vi "Status System State.vi"(5 "Retry Attempts (0)":i32 min=0, 7 "Unit Address (-1)":i32=-1, 8 "error in (no error)":errorcluster, 11 "VISA resource name (in)":refnum<visa-resource-name>) -> (0 "error out":errorcluster, 2 "System State":T1, 3 "VISA resource name (out)":refnum<visa-resource-name>)   [LabVIEW 2020, in "Omega Platinum Series.lvlib"]
doc: "Checks the current System State of the controller."
uses:
  <instrlib>/RxnRover/OmegaPlatinumSeriesDriver/Omega Platinum Series.lvlib
  <instrlib>/RxnRover/OmegaPlatinumSeriesDriver/Public/Type Defs/System State.ctl
panel:
  out "Command":string
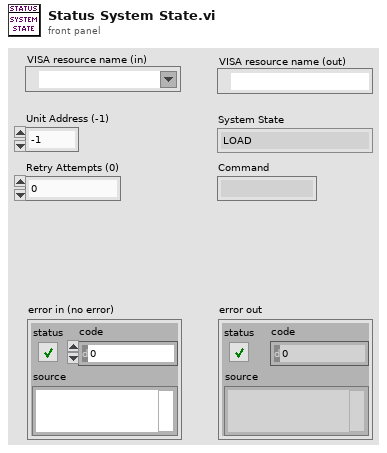
[diagram p1: front panel]
types:
  T1 = typedef "Omega Platinum Series.lvlib/System State.ctl" = enum16{"LOAD", "IDLE", "INPUT_ADJUST", "CONTROL_ADJUST", "MODIFY", "WAIT", "RUN", "STANDBY", "STOP", "PAUSE", "FAULT", "SHUTDOWN", "AUTOTUNE"}
  T2 = typedef "Omega Platinum Series.lvlib/Response.ctl" = cluster{"Unit Address":i32, "Command Class":string, "Command ID":u32, "Parameters":string}
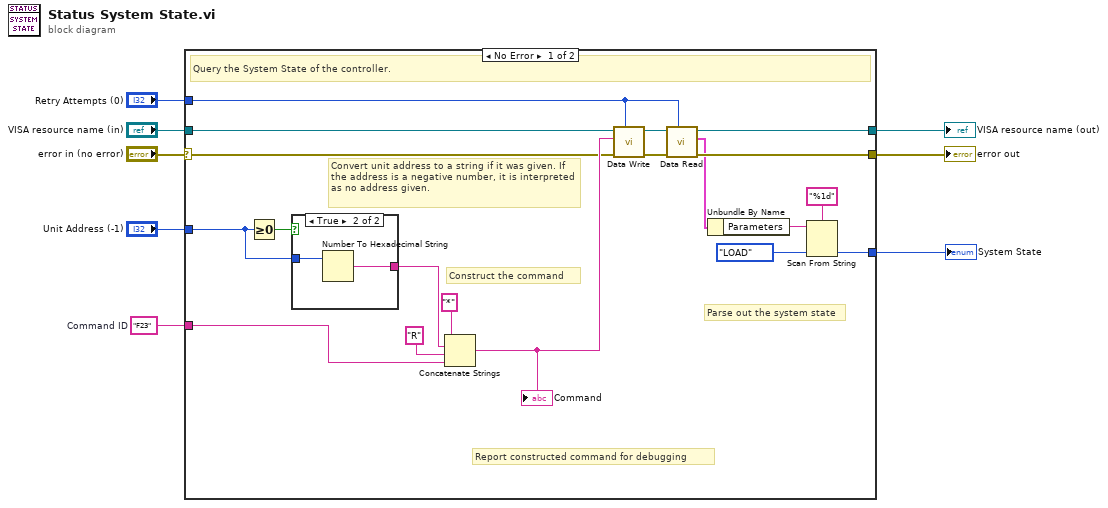
[diagram p0: block diagram]
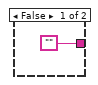
[diagram p2: hidden frame]
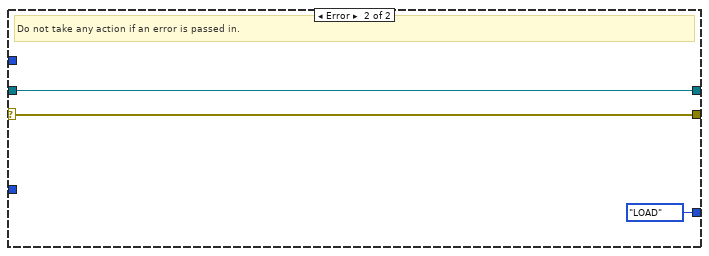
[diagram p3: hidden frame]
diagram:
  w8 = "F23"  # Command ID
  n1 = case shown="No Error" "error in (no error)" {
    selector: "error in (no error)" -> [w21 w33]
    tunnel: w8 -> [w15 _]
    tunnel: "Unit Address (-1)" -> [w25 _]
    tunnel: [w17 w33] -> w5
    tunnel: "VISA resource name (in)" -> [w23 w32]
    tunnel: [w18 w32] -> w3
    tunnel: [w10 System_State."LOAD" ("System State")] -> w2
    tunnel: "Retry Attempts (0)" -> [w9 _]
    frame No Error {
      # "Parse out the system state"
      # "Report constructed command for debugging"
      # "Convert unit address to a string if it was given. If the address is a negative number, it is interpreted as no address given."
      # "Construct the command"
      # "Query the System State of the controller."
      n2 = Greater Or Equal To 0?(x=w25) -> (x >= 0?=w27:bool)
      n3 = case shown="True" w27 {
        tunnel: w25 -> [_ w30]
        tunnel: ["" w29] -> w24
        frame False {
        }
        frame True {
          n4 = Number To Hexadecimal String(2:w30) -> (0:w29:string)  [unwired: 1 in]
        }
      }
      n5 = Concatenate Strings("*" ("string"), w24, "R" ("string"), w15) -> (w22:string)
      "Command" <- w22
      n6 = call <instrlib>:"Data Write.vi"("Retry Attempts (0)"=w9, "error in (no error)"=w21, "Command"=w22, "VISA Refnum in"=w23) -> ("error out"=w20:errorcluster, "VISA Refnum out"=w19:refnum<visa-resource-name>)  [unwired: 6 in]
      n7 = call <instrlib>:"Data Read.vi"("Retry Attempts (0)"=w9, "error in (no error)"=w20, "VISA Refnum in"=w19) -> ("error out"=w17:errorcluster, "Response Cluster"=w14:T2, "VISA Refnum out"=w18:refnum<visa-resource-name>)  [unwired: 5 in, 1 out]
      n8 = Unbundle By Name(w14) -> ("Parameters"=w13:string)
      n9 = Scan From String(format string="%1d", input string=w13, default 1=System_State."LOAD" ("System State")) -> (output 1=w10:T1)  [unwired: 2 in, 3 out]
    }
    frame Error {
      # "Do not take any action if an error is passed in."
    }
  }
  "error out" <- w5
  "VISA resource name (out)" <- w3
  "System State" <- w2
